vi "Save Time Entry.vi"(8 "error in (no error)":errorcluster, 11 "Time Entry-INI in":refnum<class "Time Entry-INI.lvclass">) -> (0 "error out":errorcluster, 3 "Time Entry-INI out":refnum<class "Time Entry-INI.lvclass">)   [LabVIEW 2020, in "Time Entry-INI.lvclass"]
doc: "VI for override that will save the specific time entry to the file/database/other specified for record keeping.\n\n04/2025 Erich Schlieper"
uses:
  Time Entry-INI.lvclass
  C:/Apps/LVTimeTracker/LVTimeTracker/Time Entries/Time Entry/Time Entries.lvclass
  Time Entry-INI.lvclass/Time Entry-INI.ctl
  <vilib>/Utility/config.llb/Write Key (String).vi
  <vilib>/Utility/config.llb/Write Key (Double).vi
  <vilib>/Utility/config.llb/NI_LVConfig.lvlib
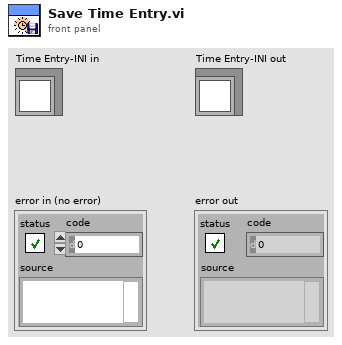
[diagram p1: front panel]
types:
  T1 = typedef "NI_LVConfig.lvlib/Config Data RefNum.ctl" = refnum<k1>
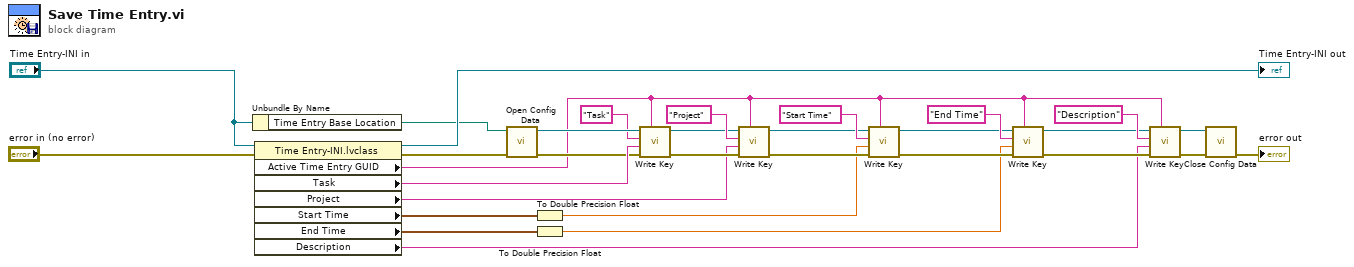
[diagram p0: block diagram]
diagram:
  n1 = Unbundle By Name("Time Entry-INI in") -> ("Time Entry Base Location"=w28:path)
  n2 = property class="Time Entry-INI.lvclass"(reference="Time Entry-INI in", error in="error in (no error)") -> (reference out=→"Time Entry-INI out":refnum<class "Time Entry-INI.lvclass">, error out=w27:errorcluster, "Active Time Entry GUID"=w18:string, "Task"=w25:string, "Project"=w9:string, "Start Time"=w8:timestamp, "End Time"=w6:timestamp, "Description"=w4:string)
  n3 = call <vilib>:"Open Config Data.vi"("error in (no error)"=w27, "configuration file path"=w28) -> ("error out"=w23:errorcluster, "refnum"=w26:T1)  [unwired: 7 in, 1 out]
  n4 = To Double Precision Float(number=w8) -> (double precision float=w7:dbl)
  n5 = To Double Precision Float(number=w6) -> (double precision float=w5:dbl)
  n6 = call-poly <vilib>:"Write Key.vi"("section"=w18, "error in (no error)"=w23, "value"=w25, "key"="Task", "refnum"=w26) -> ("error out"=w13:errorcluster, "refnum out"=w17:T1)  [unwired: 4 in, 1 out]
  n7 = call-poly <vilib>:"Write Key.vi"("section"=w18, "error in (no error)"=w13, "value"=w9, "key"="Project", "refnum"=w17) -> ("error out"=w12:errorcluster, "refnum out"=w16:T1)  [unwired: 4 in, 1 out]
  n8 = call-poly <vilib>:"Write Key.vi"("section"=w18, "error in (no error)"=w12, "value"=w7, "key"="Start Time", "refnum"=w16) -> ("error out"=w11:errorcluster, "refnum out"=w15:T1)  [unwired: 4 in, 1 out]
  n9 = call-poly <vilib>:"Write Key.vi"("section"=w18, "error in (no error)"=w11, "value"=w5, "key"="End Time", "refnum"=w15) -> ("error out"=w10:errorcluster, "refnum out"=w14:T1)  [unwired: 4 in, 1 out]
  n10 = call-poly <vilib>:"Write Key.vi"("section"=w18, "error in (no error)"=w10, "value"=w4, "key"="Description", "refnum"=w14) -> ("error out"=w3:errorcluster, "refnum out"=w2:T1)  [unwired: 4 in, 1 out]
  n11 = call <vilib>:"Close Config Data.vi"("error in (no error)"=w3, "refnum"=w2) -> ("error out"=→"error out":errorcluster)  [unwired: 8 in, 1 out]
